vi "GetHelpDir.vi"() -> (0 "help path":path)   [LabVIEW 2014]
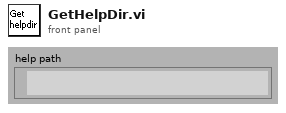
[diagram p1: front panel]
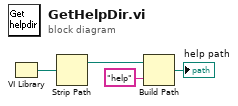
[diagram p0: block diagram]
diagram:
  n1 = VI Library() -> (path=w4:path)
  n2 = Strip Path(path=w4) -> (stripped path=w3:path)  [unwired: 1 out]
  n3 = Build Path(base path=w3, name or relative path="help") -> (appended path=→"help path":path)
